vi "CONCATINATE_STRING.vi"(9 "F-format string":string, 11 "F-format string 2":string) -> (2 "concatenated string":string)   [LabVIEW 2017]
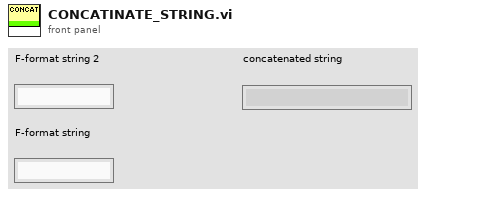
[diagram p1: front panel]
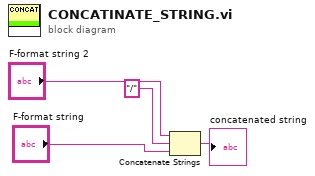
[diagram p0: block diagram]
diagram:
  n1 = Concatenate Strings("F-format string 2", "/" ("string"), "F-format string") -> (→"concatenated string":string)
